vi "Set active Layer programmatically.vi"(8 "error in":errorcluster, 9 "Active Layer []":i32[](array[numeric]), 10 "Active Layer":i32, 11 "Data in":T1={"Class"={"Ants"=refnum, "Layer"=refnum, "Templates"=refnum, "Icon"=refnum, "Glyph"=refnum, "Settings"=refnum, "Tools"=refnum}, "Ref"={"Add Layer"=refnum, "Remove Layer"=refnum, "Line Text"=[], "Body Text Spec"=refnum, "DNL_Font"=refnum, "glyph path str"=refnum, "templates path str"=refnum, "Arrow Up"=refnum, "Arrow Down"=refnum, "IE VI Ref"=refnum, "Glyphs tree"=refnum, "Templates tree"=refnum, "Layer Icon Text"=refnum, "Layer Template"=refnum, "Clipboard"=refnum, "BW icon in"=refnum, "Color icon in"=refnum, "Layer Clust"=refnum, "Body Text"=refnum, "DNL_Framework Templates"=refnum, "Search Templates"=refnum, "TextMarker"=refnum, "Tab Control"=refnum, "Search Glyphs"=refnum, "Line Color"=refnum, "DNL_Glyphs []"=refnum, "Fill Color"=refnum, "Tools"=refnum, "Glyphs tree"=refnum, "Icon"=refnum, "Preview"=refnum, "Ants"=refnum, "Terminals"=refnum, "menu reference"=refnum, "LayerNames"=[], "GlyphLoadAnimation"=refnum, "TemplateLoadAnimation"=refnum, "refreshGlyphs"=refnum, "refreshTemplates"=refnum}, "Support"={"AntsRect"={"left"=0, "top"=0, "right"=0, "bottom"=0}, "Mouse Move Coords"={"Horizontal"=0, "Vertical"=0}, "Mouse Down Coords"={"Horizontal"=0, "Vertical"=0}, "Temp Coord"={"Horizontal"=0, "Vertical"=0}, "Action"=enum."Default", "Edge Color"=4914962, "Fill Color"=16860, "Mouse Down?"=FALSE, "Draft Mode?"=FALSE, "Temp Icon"=bytes[3102], "CTRL Pressed"=FALSE, "Move Selection?"=FALSE, "AntsRect Orig"={"left"=0, "top"=0, "right"=0, "bottom"=0}, "Text"="", "TM Set?"=FALSE, "Mouse inside icon?"=FALSE, "Tool (old value)"=0, "Pencil Move Color"=0, "Swap Colors?"=FALSE, "Shift pressed?"=FALSE}}) -> (0 "error out":errorcluster, 3 "Data out":T1={"Class"={"Ants"=refnum, "Layer"=refnum, "Templates"=refnum, "Icon"=refnum, "Glyph"=refnum, "Settings"=refnum, "Tools"=refnum}, "Ref"={"Add Layer"=refnum, "Remove Layer"=refnum, "Line Text"=[], "Body Text Spec"=refnum, "DNL_Font"=refnum, "glyph path str"=refnum, "templates path str"=refnum, "Arrow Up"=refnum, "Arrow Down"=refnum, "IE VI Ref"=refnum, "Glyphs tree"=refnum, "Templates tree"=refnum, "Layer Icon Text"=refnum, "Layer Template"=refnum, "Clipboard"=refnum, "BW icon in"=refnum, "Color icon in"=refnum, "Layer Clust"=refnum, "Body Text"=refnum, "DNL_Framework Templates"=refnum, "Search Templates"=refnum, "TextMarker"=refnum, "Tab Control"=refnum, "Search Glyphs"=refnum, "Line Color"=refnum, "DNL_Glyphs []"=refnum, "Fill Color"=refnum, "Tools"=refnum, "Glyphs tree"=refnum, "Icon"=refnum, "Preview"=refnum, "Ants"=refnum, "Terminals"=refnum, "menu reference"=refnum, "LayerNames"=[], "GlyphLoadAnimation"=refnum, "TemplateLoadAnimation"=refnum, "refreshGlyphs"=refnum, "refreshTemplates"=refnum}, "Support"={"AntsRect"={"left"=0, "top"=0, "right"=0, "bottom"=0}, "Mouse Move Coords"={"Horizontal"=0, "Vertical"=0}, "Mouse Down Coords"={"Horizontal"=0, "Vertical"=0}, "Temp Coord"={"Horizontal"=0, "Vertical"=0}, "Action"=enum."Default", "Edge Color"=4914962, "Fill Color"=16860, "Mouse Down?"=FALSE, "Draft Mode?"=FALSE, "Temp Icon"=bytes[3102], "CTRL Pressed"=FALSE, "Move Selection?"=FALSE, "AntsRect Orig"={"left"=0, "top"=0, "right"=0, "bottom"=0}, "Text"="", "TM Set?"=FALSE, "Mouse inside icon?"=FALSE, "Tool (old value)"=0, "Pencil Move Color"=0, "Swap Colors?"=FALSE, "Shift pressed?"=FALSE}})   [LabVIEW 2021]
uses:
  <resource>/plugins/NIIconEditor/Controls/IE Data.ctl
  <resource>/plugins/NIIconEditor/Class/Ants/Ants.lvclass
  <resource>/plugins/NIIconEditor/Class/FakedArray/FakedArray.lvclass
  <vilib>/LabVIEW Icon API/lv_icon/Classes/Icon/Icon.lvclass
  <resource>/plugins/NIIconEditor/Class/Icon Library/Glyph.lvclass
  <resource>/plugins/NIIconEditor/Class/Settings/Settings.lvclass
  <resource>/plugins/NIIconEditor/Class/Tools/Tools Paint.lvclass
  <resource>/plugins/NIIconEditor/Controls/IE Classes.ctl
  <resource>/plugins/NIIconEditor/Controls/References Cluster.ctl
  <resource>/plugins/NIIconEditor/Controls/SupportClass.ctl
  <vilib>/Utility/miscctls.llb/LVPoint32TypeDef.ctl
  <resource>/plugins/NIIconEditor/Controls/SupportClass_Action.ctl
  <vilib>/LabVIEW Icon API/lv_icon/Controls/IEColor.ctl
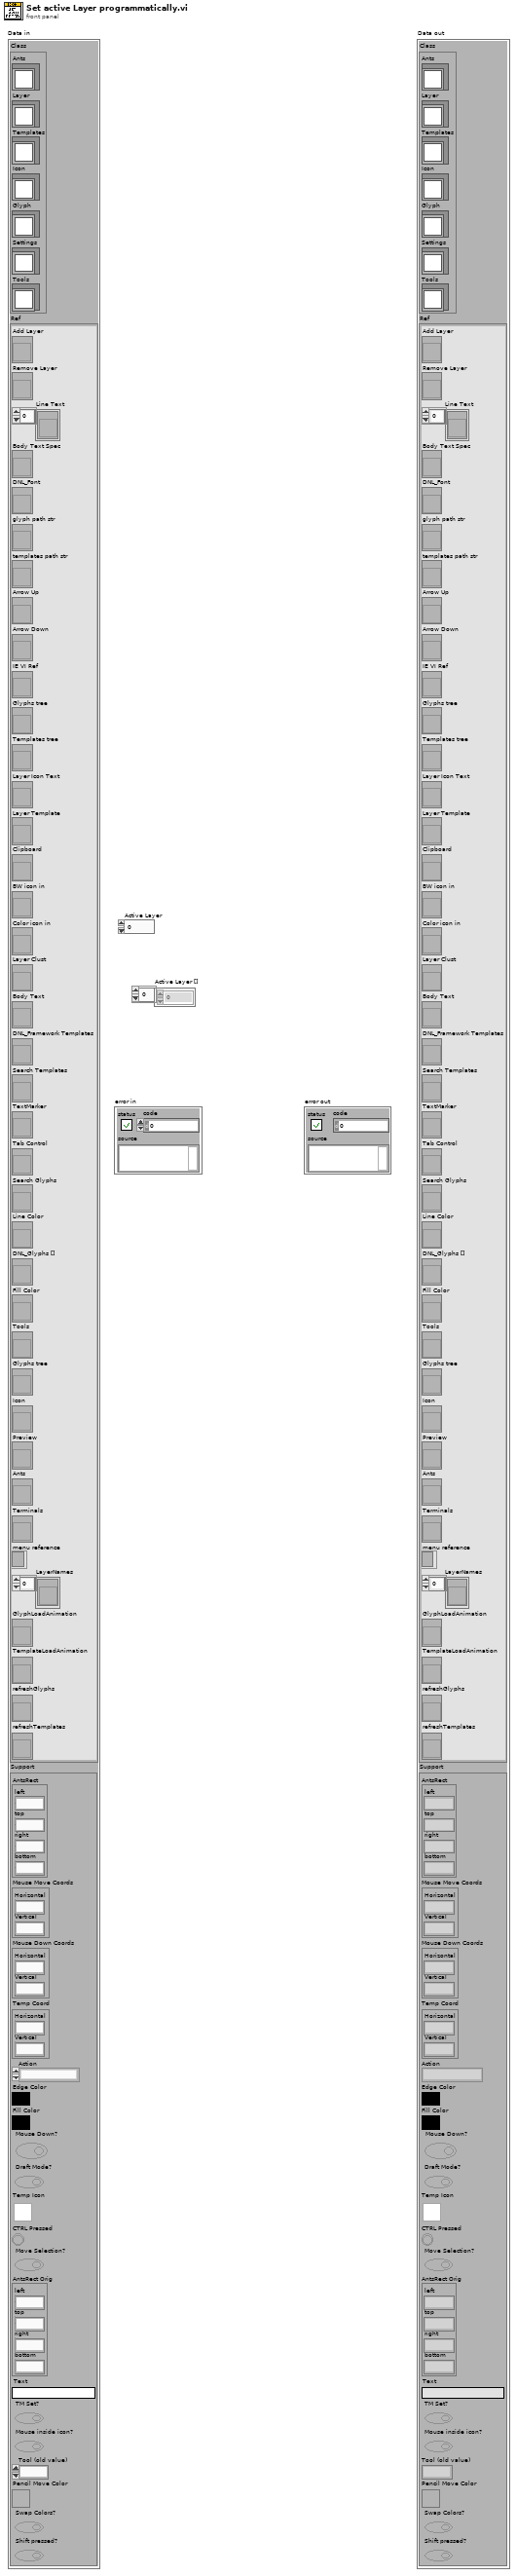
[diagram p1: front panel]
types:
  T1 = typedef "IE Data.ctl" = cluster{"Class":T2, "Ref":T3, "Support":T4}
  T2 = typedef "IE Classes.ctl" = cluster{"Ants":refnum<class "Ants.lvclass">, "Layer":refnum<class "FakedArray.lvclass">, "Templates":refnum<class "FakedArray.lvclass">, "Icon":refnum<class "Icon.lvclass">, "Glyph":refnum<class "Glyph.lvclass">, "Settings":refnum<class "Settings.lvclass">, "Tools":refnum<class "Tools Paint.lvclass">}
  T3 = typedef "References Cluster.ctl" = cluster{"Add Layer":refnum<vi>, "Remove Layer":refnum<vi>, "Line Text":refnum<vi>[], "Body Text Spec":refnum<vi>, "DNL_Font":refnum<vi>, "glyph path str":refnum<vi>, "templates path str":refnum<vi>, "Arrow Up":refnum<vi>, "Arrow Down":refnum<vi>, "IE VI Ref":refnum<vi>, "Glyphs tree":refnum<vi>, "Templates tree":refnum<vi>, "Layer Icon Text":refnum<vi>, "Layer Template":refnum<vi>, "Clipboard":refnum<vi>, "BW icon in":refnum<vi>, "Color icon in":refnum<vi>, "Layer Clust":refnum<vi>, "Body Text":refnum<vi>, "DNL_Framework Templates":refnum<vi>, "Search Templates":refnum<vi>, "TextMarker":refnum<vi>, "Tab Control":refnum<vi>, "Search Glyphs":refnum<vi>, "Line Color":refnum<vi>, "DNL_Glyphs []":refnum<vi>, "Fill Color":refnum<vi>, "Tools":refnum<vi>, "Glyphs tree":refnum<vi>, "Icon":refnum<vi>, "Preview":refnum<vi>, "Ants":refnum<vi>, "Terminals":refnum<vi>, "menu reference":refnum<k9>, "LayerNames":refnum<vi>[], "GlyphLoadAnimation":refnum<vi>, "TemplateLoadAnimation":refnum<vi>, "refreshGlyphs":refnum<vi>, "refreshTemplates":refnum<vi>}
  T4 = typedef "SupportClass.ctl" = cluster{"AntsRect":cluster{"left":i16, "top":i16, "right":i16, "bottom":i16}, "Mouse Move Coords":T5, "Mouse Down Coords":T5, "Temp Coord":T5, "Action":T6, "Edge Color":T7, "Fill Color":T7, "Mouse Down?":bool, "Draft Mode?":bool, "Temp Icon":picture, "CTRL Pressed":bool, "Move Selection?":bool, "AntsRect Orig":cluster{"left":i16, "top":i16, "right":i16, "bottom":i16}, "Text":string, "TM Set?":bool, "Mouse inside icon?":bool, "Tool (old value)":u32, "Pencil Move Color":u32, "Swap Colors?":bool, "Shift pressed?":bool}
  T5 = typedef "LVPoint32TypeDef.ctl" = cluster{"Horizontal":i32, "Vertical":i32}
  T6 = typedef "SupportClass_Action.ctl" = enum16{"Default", "Move Selection", "Glyph Library", "Tool"}
  T7 = typedef "IEColor.ctl" = u32
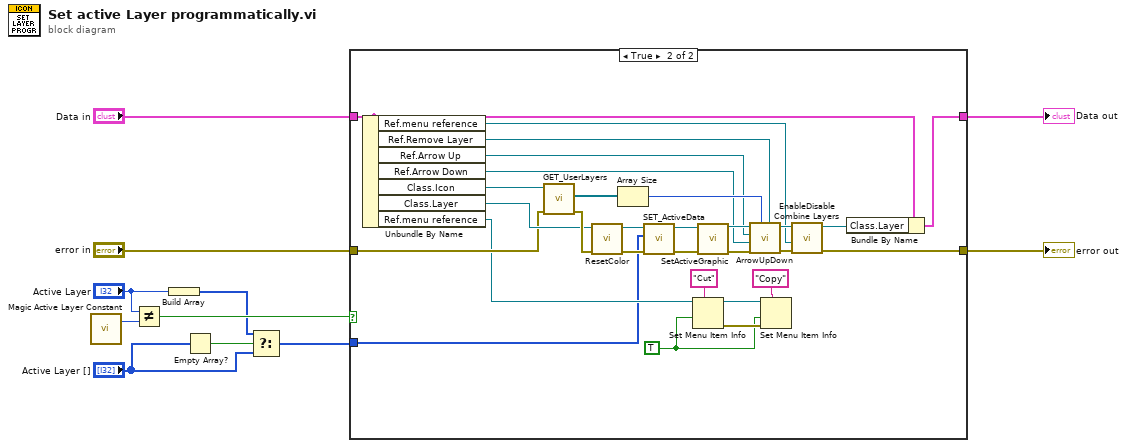
[diagram p0: block diagram]
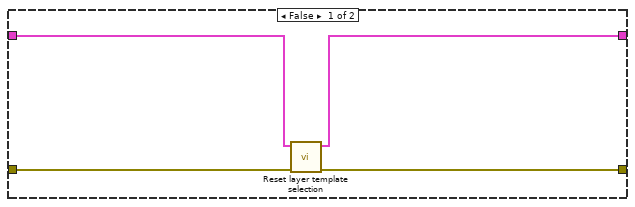
[diagram p2: hidden frame]
diagram:
  n1 = call <resource>:"Magic Active Layer Constant.vi"() -> ("Magic Constant"=w11:i32)  [unwired: 19 out]
  n2 = Not Equal?(x="Active Layer", y=w11) -> (x != y?=w10:bool)
  n3 = Build Array("Active Layer") -> (w4:i32[])
  n4 = Empty Array?(array="Active Layer []") -> (empty?=w6:bool)
  n5 = Select(t=w4, s=w6, f="Active Layer []") -> (s? t:f=w3:i32[])
  n6 = case shown="True" w10 {
    tunnel: "error in" -> [w15 w31]
    tunnel: [w14 w28] -> w2
    tunnel: "Data in" -> [w13 w30]
    tunnel: [w12 w27] -> w8
    tunnel: w3 -> [_ w16]
    frame False {
      n7 = call <resource>:"Reset layer template selection.vi"("error in (no error)"=w15, "Data in"=w13) -> ("error out"=w14:errorcluster, "Data out"=w12:T1)  [unwired: 1 in, 7 out]
    }
    frame True {
      w17 = TRUE
      n8 = Unbundle By Name(w30) -> ("Ref.menu reference"=w26:refnum<k9>, "Ref.Remove Layer"=w23:refnum<vi>, "Ref.Arrow Up"=w24:refnum<vi>, "Ref.Arrow Down"=w25:refnum<vi>, "Class.Icon"=w33:refnum<class "Icon.lvclass">, "Class.Layer"=w32:refnum<class "FakedArray.lvclass">, "Ref.menu reference"=w18:refnum<k9>)
      n9 = call-dynamic "GET_UserLayers.vi"("error in (no error)"=w31, "Icon.lvclass in"=w33) -> ("error out"=w42:errorcluster, "All Layers"=w43:refnum<class "Layer.lvclass">[])  [unwired: 8 out]
      n10 = call <resource>:"ResetColor.vi"("error in (no error)"=w42, "FakedArray in"=w32) -> ("error out"=w37:errorcluster, "FakedArray out"=w36:refnum<class "FakedArray.lvclass">)  [unwired: 8 out]
      n11 = Array Size(array=w43) -> (size(s)=w44:i32)
      n12 = call-dynamic "SET_ActiveData.vi"("error in (no error)"=w37, "Active Data"=w16, "FakedArray.lvclass in"=w36) -> ("error out"=w34:errorcluster, "FakedArray.lvclass out"=w35:refnum<class "FakedArray.lvclass">)  [unwired: 7 out]
      n13 = Set Menu Item Info(7:"Cut" ("item tag"), 9:w17, 11:w18) -> (0:w19:errorcluster, 3:w21:refnum<k9>)  [unwired: 1 in, 3 out]
      n14 = call-dynamic "SetActiveGraphic.vi"("error in (no error)"=w34, "FakedArray in"=w35) -> ("error out"=w40:errorcluster, "FakedArray out"=w41:refnum<class "FakedArray.lvclass">)  [unwired: 4 in, 4 out]
      n15 = call <resource>:"ArrowUpDown.vi"("Remove Layer"=w23, "# Layers"=w44, "error in (no error)"=w40, "Arrow Down"=w25, "Arrow Up"=w24, "FakedArray in"=w41) -> ("error out"=w39:errorcluster, "FakedArray out"=w38:refnum<class "FakedArray.lvclass">)  [unwired: 4 out]
      n16 = Set Menu Item Info(7:"Copy" ("item tag"), 8:w19, 9:w17, 11:w21) -> ()  [unwired: 5 out]
      n17 = call <resource>:"EnableDisable Combine Layers.vi"("error in"=w39, "menu reference"=w26, "Layers Cluster"=w38) -> ("error out"=w28:errorcluster, "FakedArray out"=w29:refnum<class "FakedArray.lvclass">)  [unwired: 1 in, 6 out]
      n18 = Bundle By Name(cluster=w30, "Class.Layer"=w29) -> (w27:T1)
    }
  }
  "error out" <- w2
  "Data out" <- w8
